vi "DataLog Path.vi"(8 "错误输入":errorcluster, 11 "SN":string) -> (0 "错误输出":errorcluster)   [LabVIEW 2024]
panel:
  out "array":string[](array[string])
  out "spreadsheet string":string
  out "Array":string[](array[string])
  out "path":path
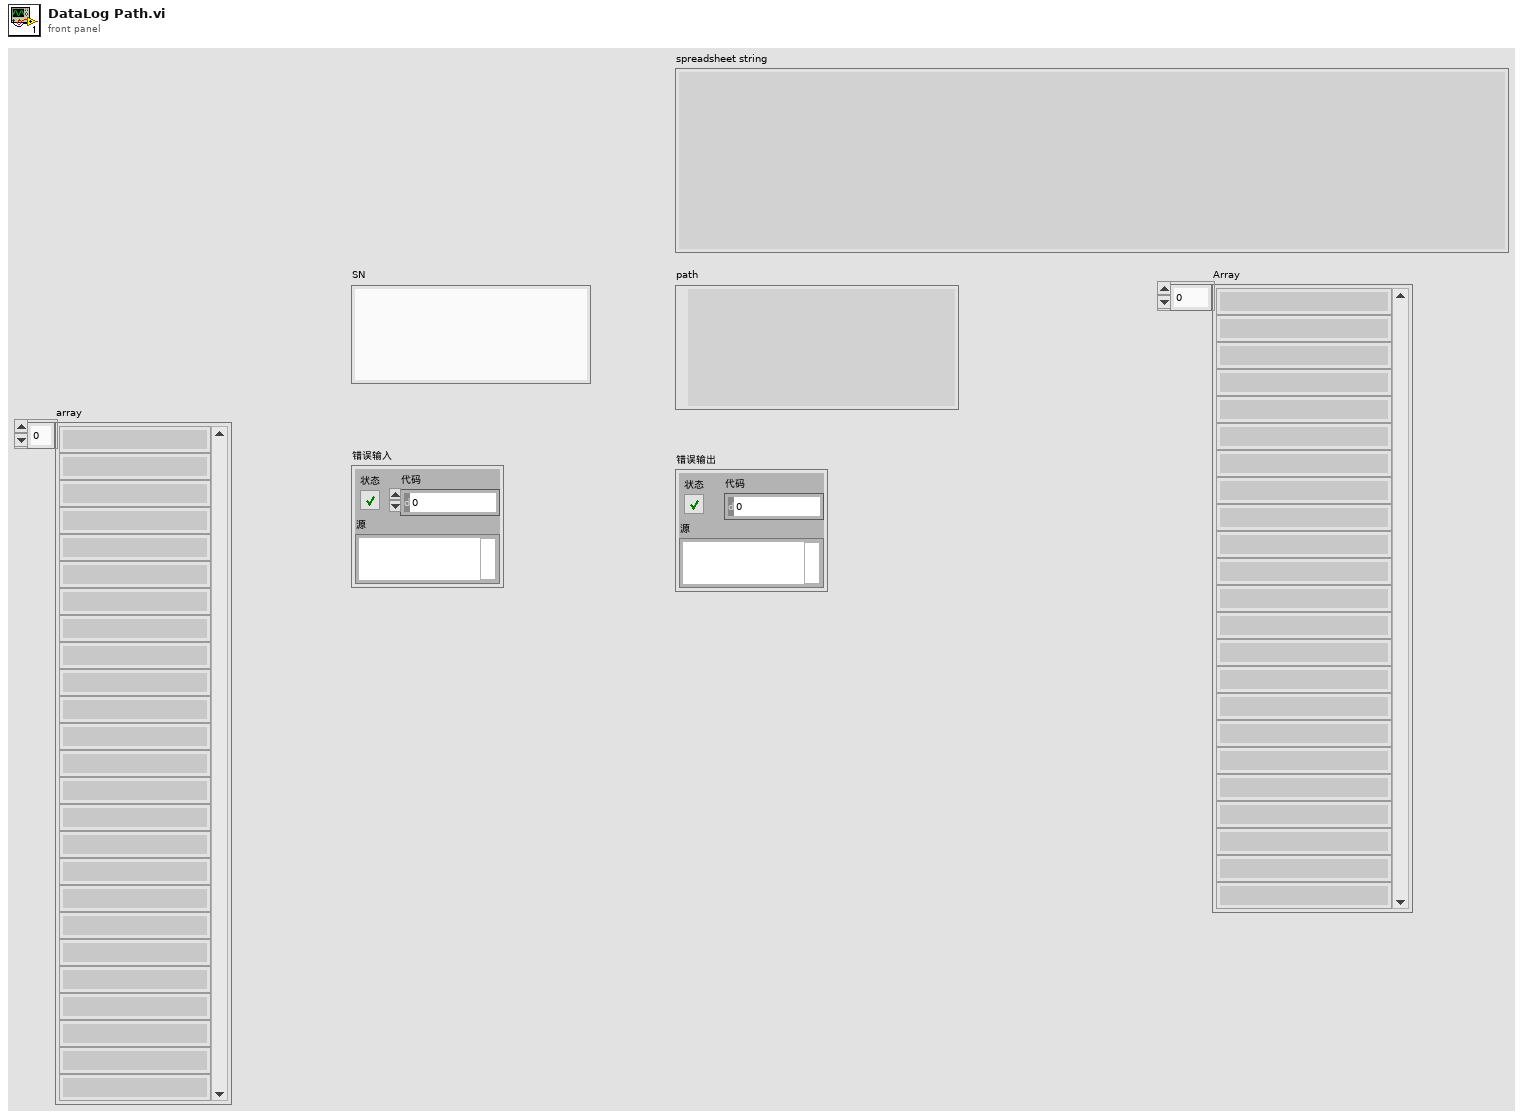
[diagram p1: front panel]
types:
  T1 = enum16{"open", "replace", "create", "open or create", "replace or create", "replace or create with confirmation"}
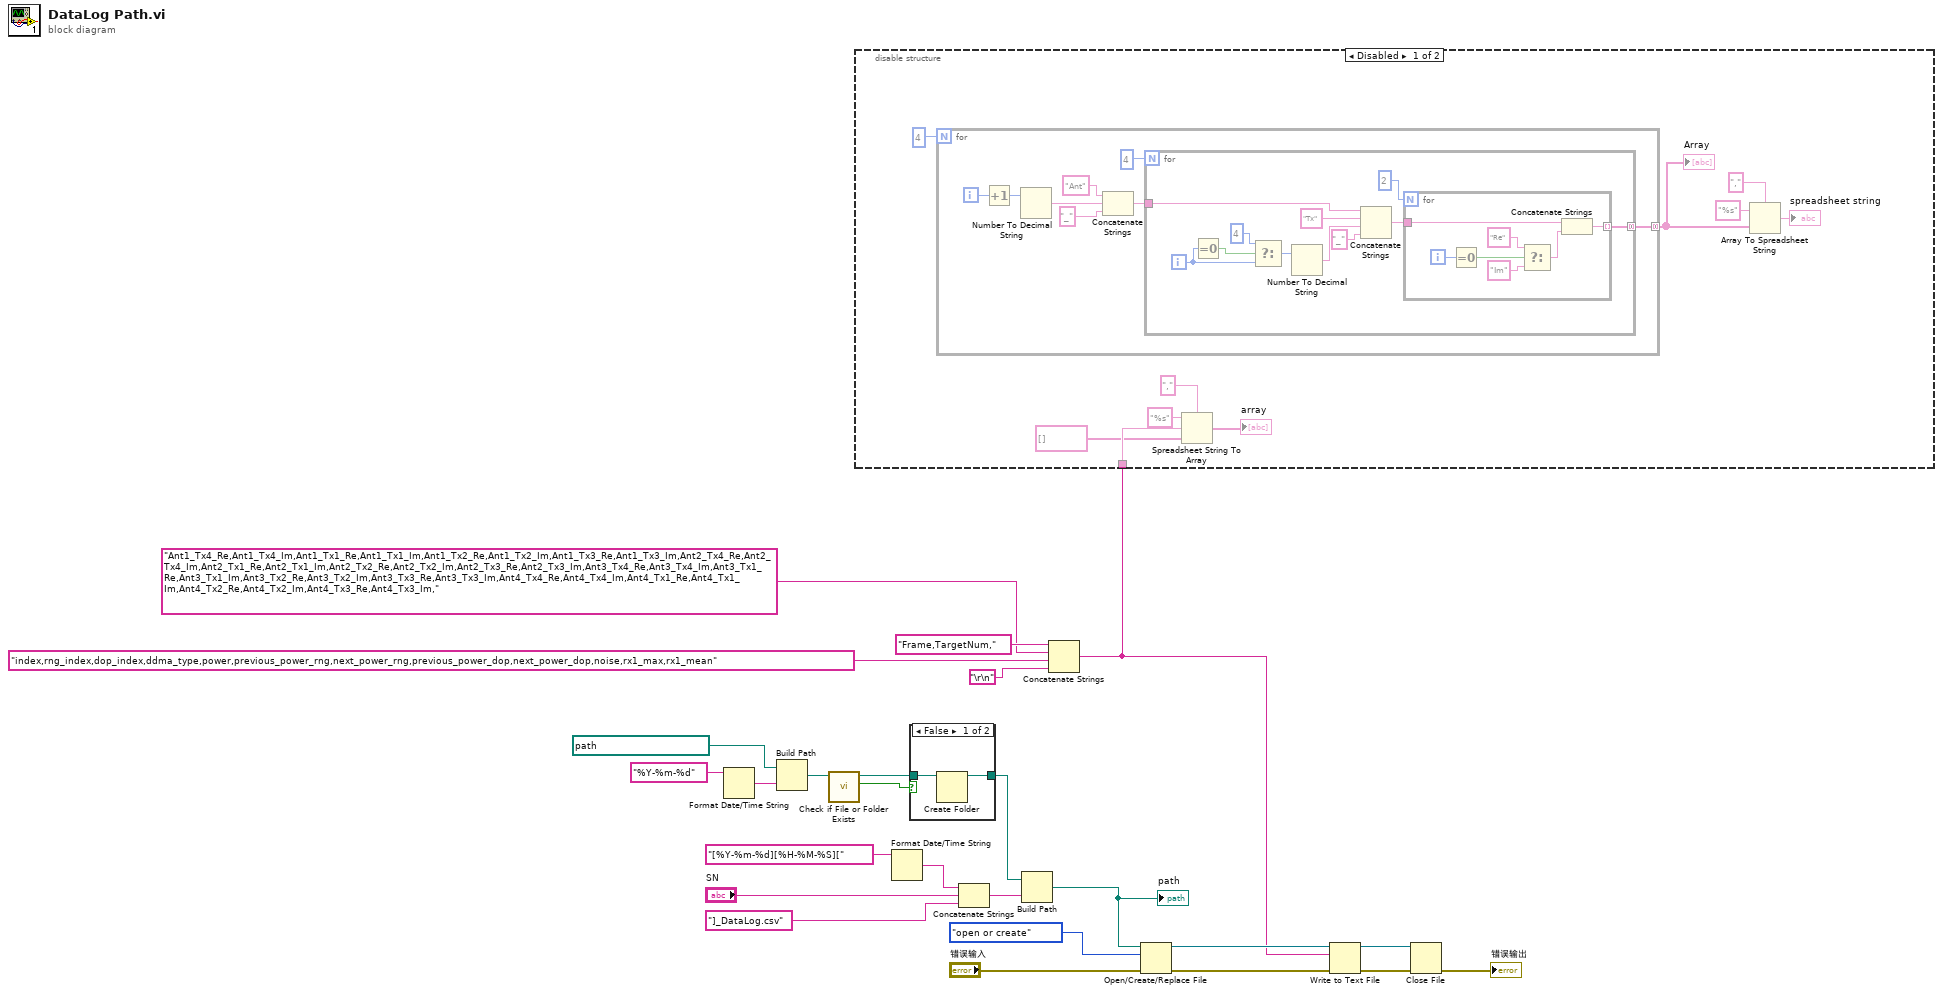
[diagram p0: block diagram]
diagram:
  n1 = Format Date/Time String(time format string (%c)="%Y-%m-%d" ("名称或相对路径")) -> (date/time string=w13:string)  [unwired: 2 in]
  n2 = Build Path(base path=path "D:/雷达测试/Data Log" ("基路径"), name or relative path=w13) -> (appended path=w23:path)
  n3 = call <vilib>:"Check if File or Folder Exists.vi"("path"=w23) -> ("file or folder exists?"=w24:bool, "dup path"=w6:path)  [unwired: 8 in, 1 out]
  n4 = Format Date/Time String(time format string (%c)="[%Y-%m-%d][%H-%M-%S][" ("时间格式字符串(%c)")) -> (date/time string=w20:string)  [unwired: 2 in]
  n5 = case shown="False" w24 {
    tunnel: w6 -> [w27 w28]
    tunnel: [w26 w28] -> w22
    frame False {
      n6 = Create Folder(path (use dialog)=w27) -> (created path=w26:path)  [unwired: 2 in, 2 out]
    }
    frame True {
    }
  }
  n7 = Concatenate Strings(w20, "SN", "]_DataLog.csv" ("字符串")) -> (w17:string)
  n8 = Build Path(base path=w22, name or relative path=w17) -> (appended path=w15:path)
  "path" <- w15
  n9 = Concatenate Strings("Frame,TargetNum,", "Ant1_Tx4_Re,Ant1_Tx4_Im,Ant1_Tx1_Re,Ant1_Tx1_Im,Ant1_Tx2_Re,Ant1_Tx2_Im,Ant1_Tx3_Re,Ant1_Tx3_Im,Ant2_Tx4_Re,Ant2_Tx4_Im,Ant2_Tx1_Re,Ant2_Tx1_Im,Ant2_Tx2_Re,Ant2_Tx2_Im,Ant2_Tx3_Re,Ant2_Tx3_Im,Ant3_Tx4_Re,Ant3_Tx4_Im,Ant3_Tx1_Re,Ant3_Tx1_Im,Ant3_Tx2_Re,Ant3_Tx2_Im,Ant3_Tx3_Re,Ant3_Tx3_Im,Ant4_Tx4_Re,Ant4_Tx4_Im,Ant4_Tx1_Re,Ant4_Tx1_Im,Ant4_Tx2_Re,Ant4_Tx2_Im,Ant4_Tx3_Re,Ant4_Tx3_Im," ("spreadsheet string 2"), "index,rng_index,dop_index,ddma_type,power,previous_power_rng,next_power_rng,previous_power_dop,next_power_dop,noise,rx1_max,rx1_mean", "\r\n") -> (w1:string)
  n10 = disable-structure shown="Disabled" {
    disable-tunnel: w1 -> [w33 _]
    frame Disabled {
      n11 = for {
        N: 4 -> [_]
        tunnel: [w40] -> w37 mode=concatenating
        i -> [w44]
        n12 = Increment(x=w44) -> (x+1=w43:i32)
        n13 = Number To Decimal String(number=w43) -> (decimal integer string=w42:string)  [unwired: 1 in]
        n14 = Concatenate Strings("Ant", w42, "_" ("string")) -> (w45:string)
        n15 = for {
          N: 4 -> [_]
          tunnel: w45 -> [w48]
          tunnel: [w50] -> w40 mode=concatenating
          i -> [w53]
          n16 = Equal To 0?(x=w53) -> (x = 0?=w55:bool)
          n17 = Select(t=4, s=w55, f=w53) -> (s? t:f=w56:i32)
          n18 = Number To Decimal String(number=w56) -> (decimal integer string=w52:string)  [unwired: 1 in]
          n19 = Concatenate Strings(w48, "Tx" ("string"), w52, "_" ("string")) -> (w47:string)
          n20 = for {
            N: 2 -> [_]
            tunnel: w47 -> [w60]
            tunnel: [w59] -> w50 mode=indexing
            i -> [w58]
            n21 = Equal To 0?(x=w58) -> (x = 0?=w64:bool)
            n22 = Select(t="Re", s=w64, f="Im") -> (s? t:f=w61:string)
            n23 = Concatenate Strings(w60, w61) -> (w59:string)
          }
        }
      }
      "Array" <- w37
      n24 = Spreadsheet String To Array(delimiter (Tab)=",", format string="%s", spreadsheet string=w33, array type (2D Dbl)=string[] []) -> (array=→"array":string[])
      n25 = Array To Spreadsheet String(delimiter (Tab)=",", array=w37, 3:"%s" ("format string")) -> (spreadsheet string=→"spreadsheet string":string)
    }
    frame Enabled {
    }
  }
  n26 = Open/Create/Replace File(file path (use dialog)=w15, error in="错误输入", operation (0:open)=T1."open or create" ("操作(0:open)")) -> (refnum out=w10:refnum<file>, error out=w9:errorcluster)  [unwired: 3 in, 1 out]
  n27 = Write to Text File(file (use dialog)=w10, text=w1, error in=w9) -> (refnum out=w7:refnum<file>, error out=w8:errorcluster)  [unwired: 1 in, 1 out]
  n28 = Close File(refnum=w7, error in=w8) -> (error out=→"错误输出":errorcluster)  [unwired: 1 out]
